vi "ConvertRegToReadData.vi"(0 "register values 0-20":u16[](array[numeric])) -> (4 "data value":T1)   [LabVIEW 2019, in "ModbusSp.lvclass"]
uses:
  ModbusSp.lvclass
  ReadData.ctl
  Modbus Data Type Conversation/Modbus DataType Conversation.lvlib
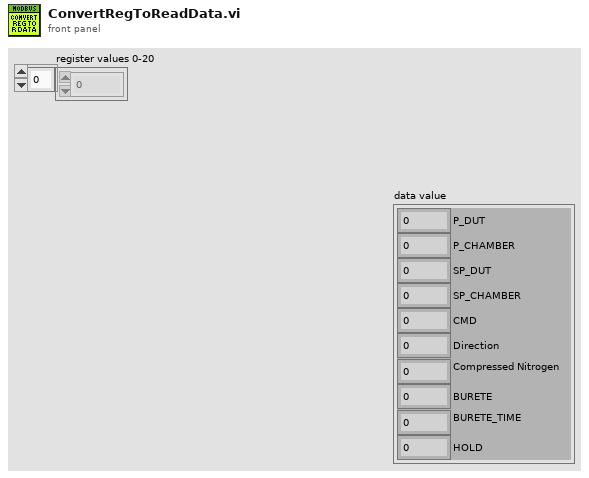
[diagram p1: front panel]
types:
  T1 = typedef "ModbusSp.lvclass/ReadData.ctl" = cluster{"P_DUT":sgl, "P_CHAMBER":sgl, "SP_DUT":sgl, "SP_CHAMBER":sgl, "CMD":u16, "Direction":u16, "Compressed Nitrogen":u16, "BURETE":u16, "BURETE_TIME":u16, "HOLD":u16}
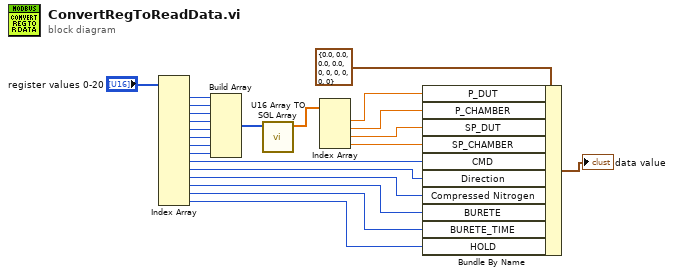
[diagram p0: block diagram]
diagram:
  n1 = Index Array(array="register values 0-20") -> (element #1=w20:u16, element #2=w19:u16, element #3=w18:u16, element #4=w17:u16, element #5=w16:u16, element #6=w15:u16, element #7=w14:u16, element #8=w13:u16, element #9=w6:u16, element #10=w5:u16, element #11=w4:u16, element #12=w3:u16, element #13=w2:u16, element #14=w1:u16)  [unwired: 14 in]
  n2 = Build Array(w20, w19, w18, w17, w16, w15, w14, w13) -> (w12:u16[])
  n3 = call "U16 Array TO SGL Array.vi"("REG U16"=w12) -> ("SGL"=w11:sgl[])  [unwired: 10 in]
  n4 = Index Array(array=w11) -> (element #1=w10:sgl, element #2=w9:sgl, element #3=w8:sgl, element #4=w7:sgl)  [unwired: 4 in]
  n5 = Bundle By Name(cluster=T1 {"P_DUT"=0.0, "P_CHAMBER"=0.0, "SP_DUT"=0.0, "SP_CHAMBER"=0.0, "CMD"=0, "Direction"=0, "Compressed Nitrogen"=0, "BURETE"=0, "BURETE_TIME"=0, "HOLD"=0} ("data value"), "P_DUT"=w10, "P_CHAMBER"=w9, "SP_DUT"=w8, "SP_CHAMBER"=w7, "CMD"=w6, "Direction"=w5, "Compressed Nitrogen"=w4, "BURETE"=w3, "BURETE_TIME"=w2, "HOLD"=w1) -> (→"data value":T1)
